vi "FPGA_counter.vi"(0 "Count or Not?":bool, 6 "Reset Photon Count":bool) -> (7 "Total Count":u8)   [LabVIEW 2024]
panel:
  # "Increment Counter if Count Or Not is true\nReset counter if Reset Photon Count changes to true"
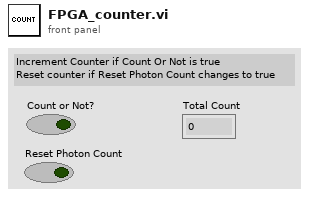
[diagram p1: front panel]
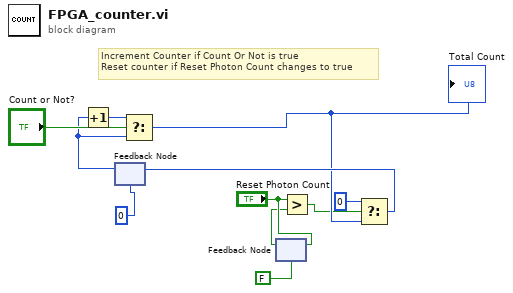
[diagram p0: block diagram]
diagram:
  # "Increment Counter if Count Or Not is true\nReset counter if Reset Photon Count changes to true"
  n1 = feedback #1(u8 0) -> (w2:u8)
  n2 = Increment(x=w2) -> (x+1=w1:u8)
  n3 = Select(t=w1, s="Count or Not?", f=w2) -> (s? t:f=w9:u8)
  "Total Count" <- w9
  n4 = feedback #2(FALSE) -> (w6:bool)
  n5 = feedback-in #2("Reset Photon Count") -> ()
  n6 = Greater?(x="Reset Photon Count", y=w6) -> (0:w8:bool)
  n7 = Select(t=u8 0, s=w8, f=w9) -> (s? t:f=w11:u8)
  n8 = feedback-in #1(w11) -> ()
